vi "Release System.vi"(8 "error in (no error)":errorcluster) -> (0 "error out":errorcluster)   [LabVIEW 2016, in "System.lvlib"]
uses:
  System.lvlib
  Controls/Control_Data Functions.ctl
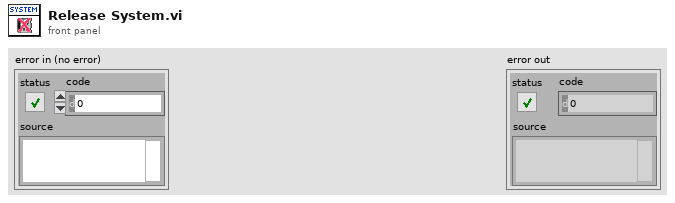
[diagram p1: front panel]
types:
  T1 = typedef "System.lvlib/Control_Data Functions.ctl" = enum16{"Get", "Set", "Release"}
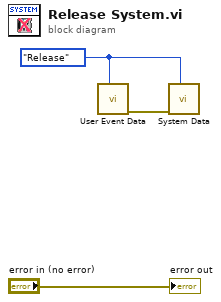
[diagram p0: block diagram]
diagram:
  w2 = Control_Data_Functions."Release" ("Data Functions")
  n1 = call "User Event Data.vi"("Data Functions"=w2) -> ("error out"=w3:errorcluster)  [unwired: 9 in, 1 out]
  n2 = call "System Data.vi"("Data Functions"=w2, "error in (no error)"=w3) -> ()  [unwired: 8 in, 2 out]
  "error out" <- "error in (no error)"
